vi "Create VI Refs.vi"(6 "Name":string, 8 "error in":errorcluster, 9 "Name Library File Path":path, 10 "Active Project":refnum<vi>) -> (0 "error out":errorcluster, 2 "VI Refs":T1)   [LabVIEW 2025, in "_Msg Rescript.lvlib" / "_Msg Rescript.lvclass"]
uses:
  _Msg Rescript.lvclass
  VI Refs.ctl
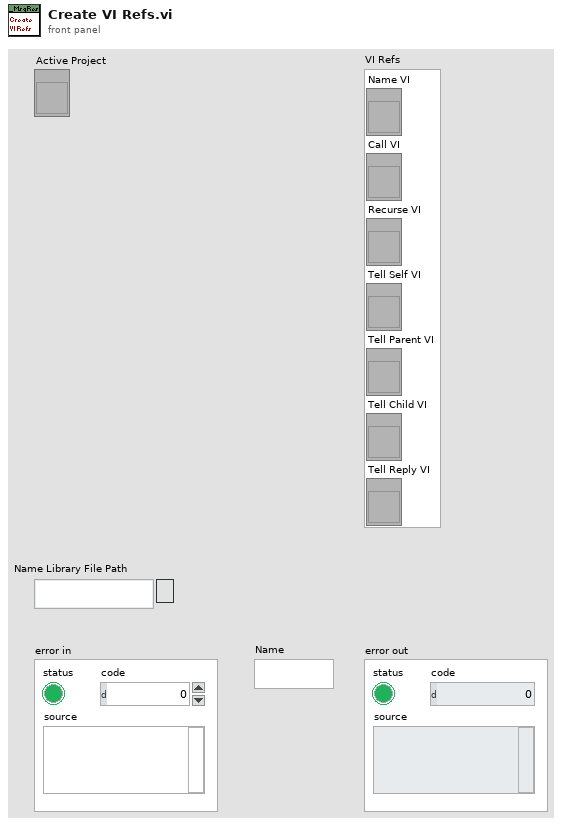
[diagram p1: front panel]
types:
  T1 = typedef "_Msg Rescript.lvlib/_Msg Rescript.lvclass/VI Refs.ctl" = cluster{"Name VI":refnum<vi>, "Call VI":refnum<vi>, "Recurse VI":refnum<vi>, "Tell Self VI":refnum<vi>, "Tell Parent VI":refnum<vi>, "Tell Child VI":refnum<vi>, "Tell Reply VI":refnum<vi>}
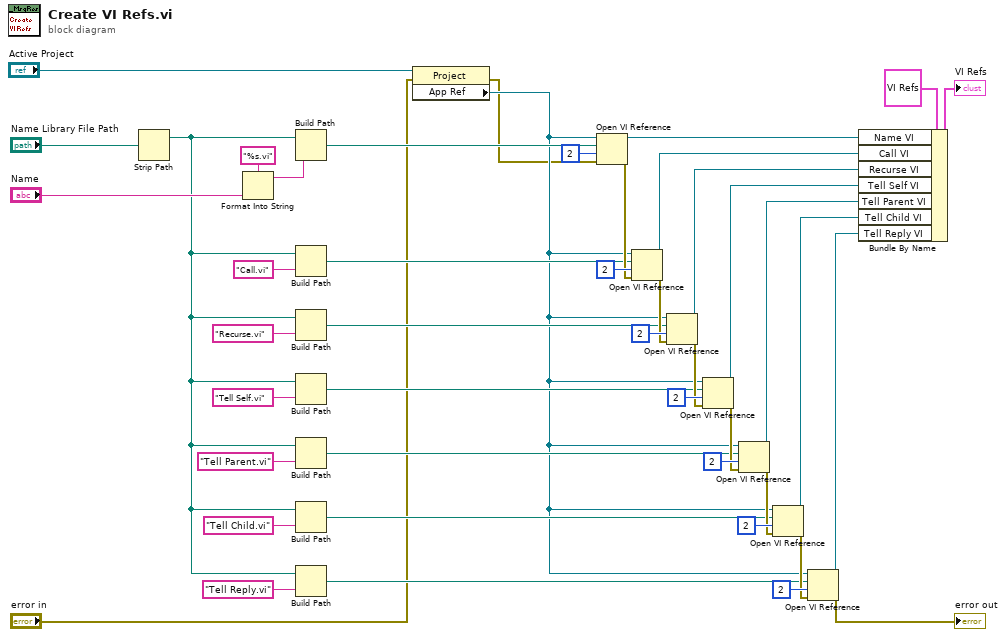
[diagram p0: block diagram]
diagram:
  n1 = Strip Path(path="Name Library File Path") -> (stripped path=w15:path)  [unwired: 1 out]
  n2 = Format Into String(format string="%s.vi", "Name") -> (resulting string=w44:string)  [unwired: 2 in, 1 out]
  n3 = Build Path(base path=w15, name or relative path=w44) -> (appended path=w43:path)
  n4 = Build Path(base path=w15, name or relative path="Call.vi" ("format string")) -> (appended path=w24:path)
  n5 = Build Path(base path=w15, name or relative path="Recurse.vi" ("format string")) -> (appended path=w23:path)
  n6 = Build Path(base path=w15, name or relative path="Tell Self.vi" ("format string")) -> (appended path=w22:path)
  n7 = Build Path(base path=w15, name or relative path="Tell Parent.vi" ("format string")) -> (appended path=w21:path)
  n8 = Build Path(base path=w15, name or relative path="Tell Child.vi" ("format string")) -> (appended path=w20:path)
  n9 = Build Path(base path=w15, name or relative path="Tell Reply.vi" ("format string")) -> (appended path=w14:path)
  n10 = property class="Project"(reference="Active Project", error in="error in") -> (error out=w1:errorcluster, "App Ref"=w3:refnum<vi>)  [unwired: 1 out]
  n11 = Open VI Reference(application reference (local)=w3, vi path=w43, options=2, error in (no error)=w1) -> (vi reference=w11:refnum<vi>, error out=w34:errorcluster)  [unwired: 2 in]
  n12 = Open VI Reference(application reference (local)=w3, vi path=w24, options=2, error in (no error)=w34) -> (vi reference=w10:refnum<vi>, error out=w33:errorcluster)  [unwired: 2 in]
  n13 = Open VI Reference(application reference (local)=w3, vi path=w23, options=2, error in (no error)=w33) -> (vi reference=w9:refnum<vi>, error out=w32:errorcluster)  [unwired: 2 in]
  n14 = Open VI Reference(application reference (local)=w3, vi path=w22, options=2, error in (no error)=w32) -> (vi reference=w8:refnum<vi>, error out=w31:errorcluster)  [unwired: 2 in]
  n15 = Open VI Reference(application reference (local)=w3, vi path=w21, options=2, error in (no error)=w31) -> (vi reference=w7:refnum<vi>, error out=w30:errorcluster)  [unwired: 2 in]
  n16 = Open VI Reference(application reference (local)=w3, vi path=w20, options=2, error in (no error)=w30) -> (vi reference=w6:refnum<vi>, error out=w17:errorcluster)  [unwired: 2 in]
  n17 = Open VI Reference(application reference (local)=w3, vi path=w14, options=2, error in (no error)=w17) -> (vi reference=w5:refnum<vi>, error out=→"error out":errorcluster)  [unwired: 2 in]
  n18 = Bundle By Name(cluster=T1 {"Name VI"=refnum, "Call VI"=refnum, "Recurse VI"=refnum, "Tell Self VI"=refnum, "Tell Parent VI"=refnum, "Tell Child VI"=refnum, "Tell Reply VI"=refnum} ("VI Refs"), "Name VI"=w11, "Call VI"=w10, "Recurse VI"=w9, "Tell Self VI"=w8, "Tell Parent VI"=w7, "Tell Child VI"=w6, "Tell Reply VI"=w5) -> (→"VI Refs":T1)
